vi "Start Tasks.vi"(8 "error in":errorcluster, 11 "cCRDS in":refnum<class "cCRDS.lvclass">=refnum) -> (0 "error out":errorcluster, 3 "cCRDS out":refnum<class "cCRDS.lvclass">)   [LabVIEW 2015, in "cCRDS.lvclass"]
uses:
  cCRDS.lvclass
  cCRDS.lvclass/cCRDS.ctl
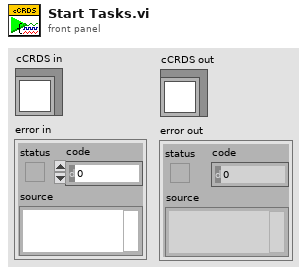
[diagram p1: front panel]
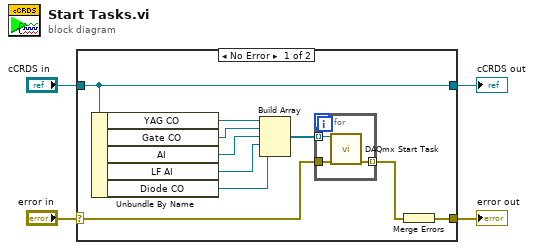
[diagram p0: block diagram]
diagram:
  n1 = case shown="No Error" "error in" {
    selector: "error in" -> [w5 w19]
    tunnel: [w12 w19] -> w3
    tunnel: [w10 w18] -> w1
    tunnel: "cCRDS in" -> [w10 w18]
    frame No Error {
      n2 = Unbundle By Name(w10) -> ("YAG CO"=w11:refnum<k21>, "Gate CO"=w9:refnum<k21>, "AI"=w8:refnum<k21>, "LF AI"=w7:refnum<k21>, "Diode CO"=w6:refnum<k21>)
      n3 = Build Array(w11, w9, w8, w7, w6) -> (w14:refnum<k21>[])
      n4 = for {
        tunnel: w14 -> [w17] mode=indexing
        tunnel: [w16] -> w13 mode=indexing
        tunnel: w5 -> [w15]
        n5 = call <vilib>:"DAQmx Start Task.vi"("task/channels in"=w17, "error in"=w15) -> ("error out"=w16:errorcluster)  [unwired: 12 in, 1 out]
      }
      n6 = Merge Errors(w13) -> (w12:errorcluster)
    }
    frame Error {
    }
  }
  "error out" <- w3
  "cCRDS out" <- w1
